vi "generujListe.vi"(10 "Plaszczyzny":i32, 11 "Punkty":i32) -> (2 "Blad":bool, 3 "Lista punktow pomiarowych":i32[][](array[numeric]))   [LabVIEW 2014]
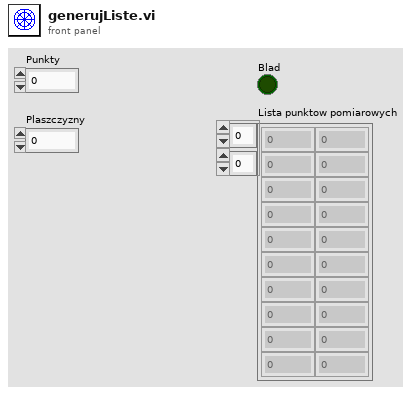
[diagram p1: front panel]
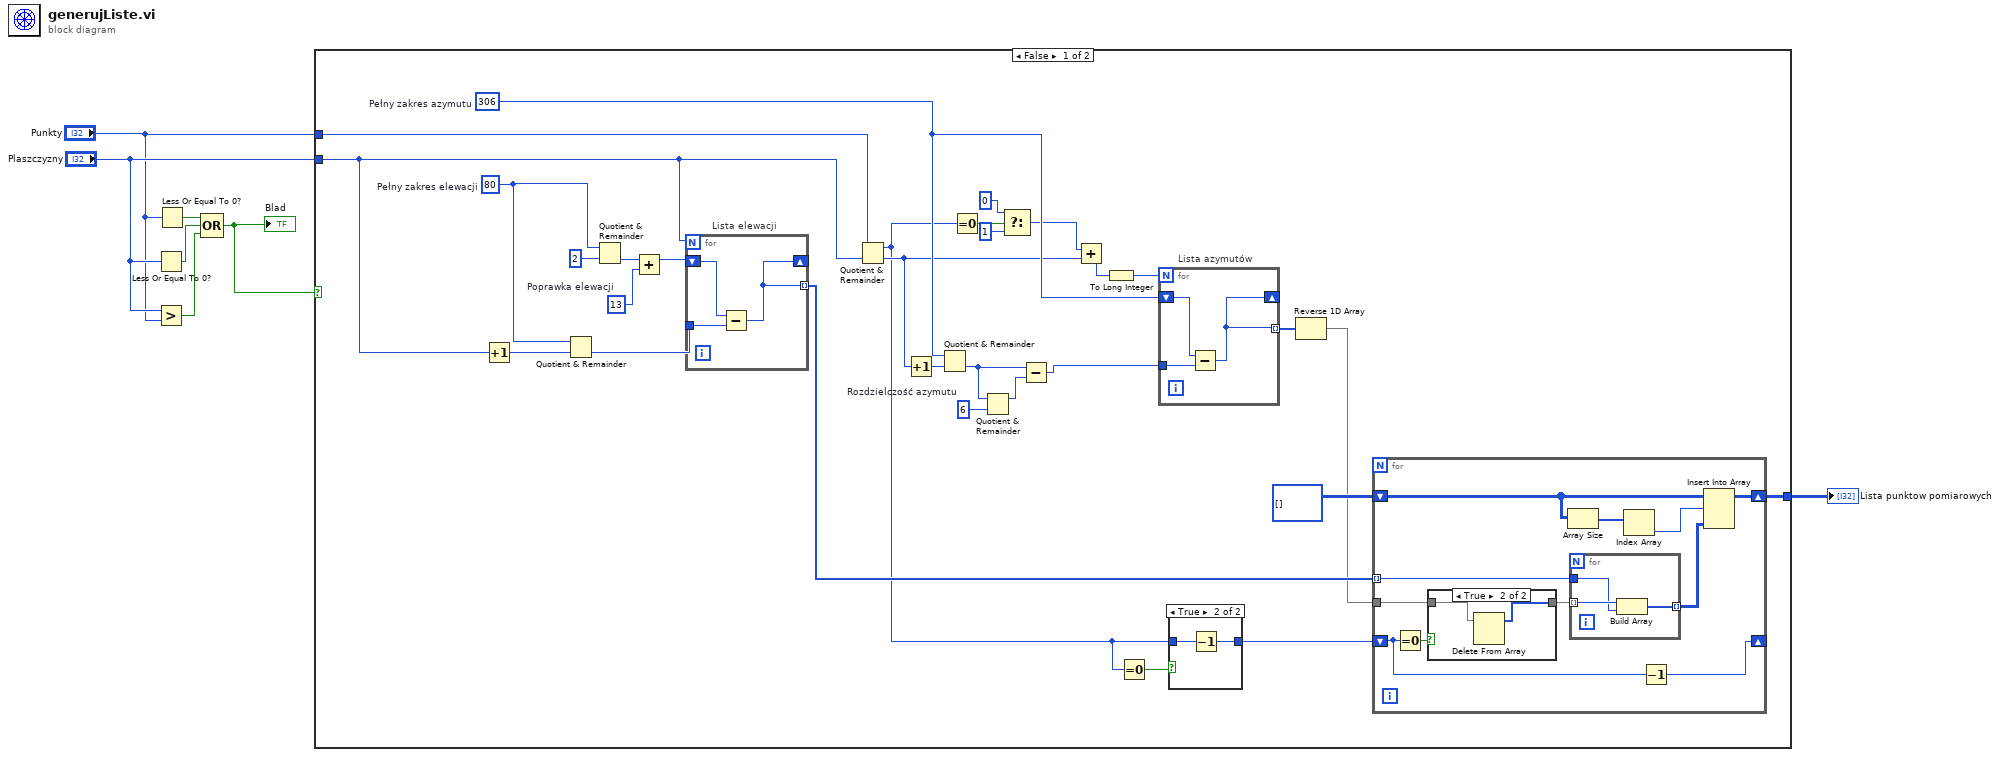
[diagram p0: block diagram]
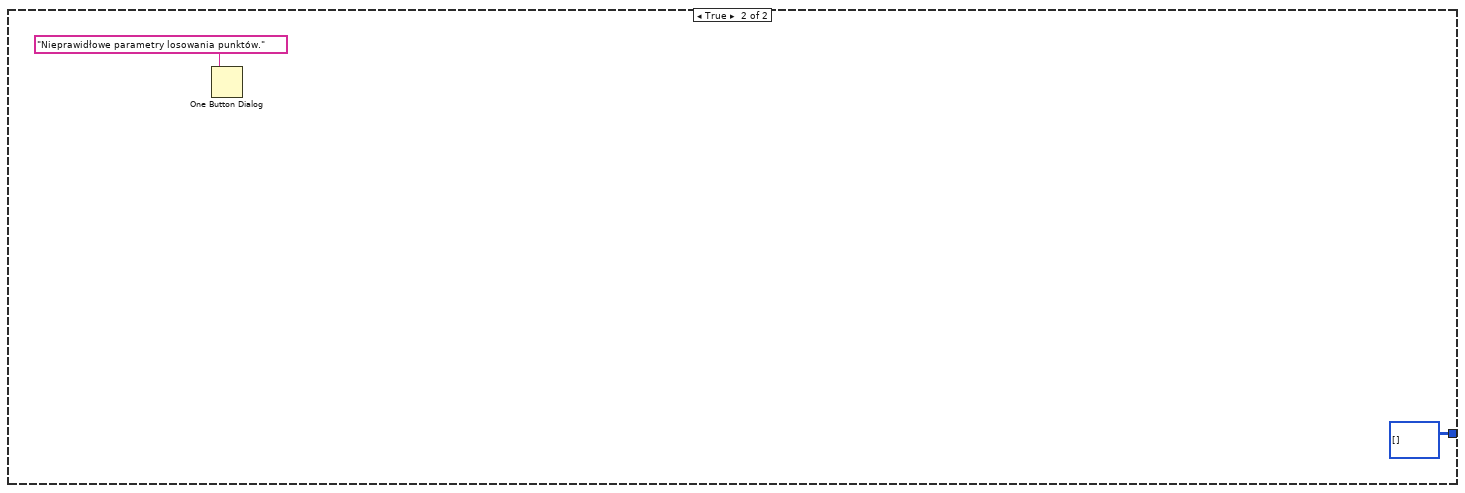
[diagram p4: hidden frame]
diagram:
  n1 = Less Or Equal To 0?(x="Plaszczyzny") -> (x <= 0?=w5:bool)
  n2 = Greater?(x="Plaszczyzny", y="Punkty") -> (0:w2:bool)
  n3 = Less Or Equal To 0?(x="Punkty") -> (x <= 0?=w6:bool)
  n4 = Compound Arithmetic op=OR(w6, w5, w2) -> (w1:bool)
  "Blad" <- w1
  n5 = case shown="False" w1 {
    tunnel: [w32 i32[][] [] ("Lista punktow pomiarowych")] -> w7
    tunnel: "Plaszczyzny" -> [w9 _]
    tunnel: "Punkty" -> [w8 _]
    frame False {
      w14 = 6  # Rozdzielczość azymutu
      w26 = 13  # Poprawka elewacji
      w35 = 306  # Pełny zakres azymutu
      w29 = 80  # Pełny zakres elewacji
      n6 = Increment(x=w9) -> (x+1=w31:i32)
      n7 = Quotient & Remainder(x=w29, y=w31) -> (floor(x/y)=w37:i32)  [unwired: 1 out]
      n8 = Quotient & Remainder(x=w29, y=2) -> (floor(x/y)=w28:i32)  [unwired: 1 out]
      n9 = Add(x=w28, y=w26) -> (x+y=w27:i32)
      n10 = for "Lista elewacji" {
        N: w9 -> [_]
        shift-right: [w61] -> _
        shift-left: w27 -> [w62]
        tunnel: w37 -> [w63]
        tunnel: [w61] -> w34 mode=indexing
        n11 = Subtract(x=w62, y=w63) -> (x-y=w61:i32)
      }
      n12 = Quotient & Remainder(x=w8, y=w9) -> (x-y*floor(x/y)=w16:i32, floor(x/y)=w23:i32)
      n13 = Increment(x=w23) -> (x+1=w36:i32)
      n14 = Quotient & Remainder(x=w35, y=w36) -> (floor(x/y)=w13:i32)  [unwired: 1 out]
      n15 = Equal To 0?(x=w16) -> (x = 0?=w21:bool)
      n16 = Quotient & Remainder(x=w13, y=w14) -> (x-y*floor(x/y)=w12:i32)  [unwired: 1 out]
      n17 = Select(t=0, s=w21, f=1) -> (s? t:f=w20:i32)
      n18 = Subtract(x=w13, y=w12) -> (x-y=w11:i32)
      n19 = Add(x=w20, y=w23) -> (x+y=w22:i32)
      n20 = To Long Integer(number=w22) -> (32bit integer=w10:i32)
      n21 = Equal To 0?(x=w16) -> (x = 0?=w17:bool)
      n22 = for "Lista azymutów" {
        N: w10 -> [_]
        shift-right: [w58] -> _
        shift-left: w35 -> [w59]
        tunnel: w11 -> [w60]
        tunnel: [w58] -> w25 mode=indexing
        n23 = Subtract(x=w59, y=w60) -> (x-y=w58:i32)
      }
      n24 = case shown="True" w17 {
        tunnel: w16 -> [w38 w40]
        tunnel: [w38 w39] -> w15
        frame False {
        }
        frame True {
          n25 = Decrement(x=w40) -> (x-1=w39:i32)
        }
      }
      n26 = Reverse 1D Array(array=w25) -> (reversed array=w24:i32[])
      n27 = for {
        tunnel: w34 -> [w51] mode=indexing
        tunnel: w24 -> [w45]
        shift-right: [w50] -> w32
        shift-left: i32[][] [] ("Lista punktow pomiarowych") -> [w48]
        shift-right: [w41] -> _
        shift-left: w15 -> [w42]
        n28 = Equal To 0?(x=w42) -> (x = 0?=w44:bool)
        n29 = case shown="True" w44 {
          tunnel: w45 -> [w52 w54]
          tunnel: [w52 w53] -> w43
          frame False {
          }
          frame True {
            n30 = Delete From Array(array=w54) -> (array with subset deleted=w53:i32[])  [unwired: 2 in, 1 out]
          }
        }
        n31 = Array Size(array=w48) -> (size(s)=w47:i32[])
        n32 = for {
          tunnel: w43 -> [w57] mode=indexing
          tunnel: w51 -> [w56]
          tunnel: [w55] -> w49 mode=indexing
          n33 = Build Array(w57, w56) -> (w55:i32[])
        }
        n34 = Index Array(array=w47) -> (element=w46:i32)  [unwired: 1 in]
        n35 = Decrement(x=w42) -> (x-1=w41:i32)
        n36 = Insert Into Array(array=w48, index (row)=w46, new element=w49) -> (w50:i32[][])  [unwired: 1 in]
      }
    }
    frame True {
      n37 = One Button Dialog(message="Nieprawidłowe parametry losowania punktów.") -> ()  [unwired: 1 in, 1 out]
    }
  }
  "Lista punktow pomiarowych" <- w7
